vi "BIO_get_ssl.vi"(8 "error in (no error)":errorcluster, 11 "BIO in":refnum<class "BIO.lvclass">) -> (0 "error out":errorcluster, 2 "SSL out":refnum<class "SSL.lvclass">, 3 "BIO out":refnum<class "BIO.lvclass">)   [LabVIEW 2013, in "OpenSSL Socket.lvlib" / "BIO.lvclass"]
uses:
  BIO.lvclass
  SSL/SSL.lvclass
  SSL-Lib/SSL-Lib.lvclass/SSL-Lib.ctl
  BIO.lvclass/BIO.ctl
  SSL/SSL.lvclass/SSL.ctl
  SSL-Lib/Read Crypto Library Path.vi
  Read Handle.vi
  SSL/Write Handle.vi
  SSL-Lib/SSL-Lib.lvclass
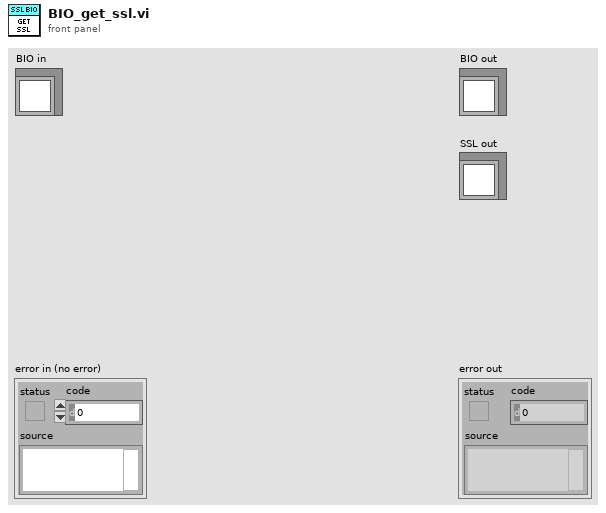
[diagram p1: front panel]
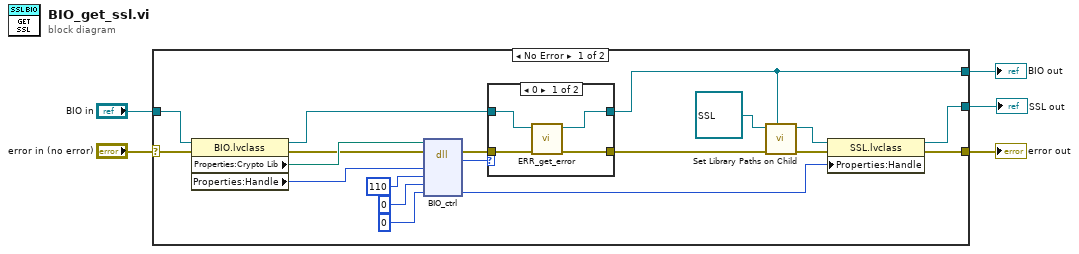
[diagram p0: block diagram]
diagram:
  n1 = case shown="No Error" "error in (no error)" {
    selector: "error in (no error)" -> [w20 w32]
    tunnel: [w7 w32] -> w4
    tunnel: [w10 w31] -> w2
    tunnel: "BIO in" -> [w21 w31]
    tunnel: [w6 _] -> w1
    frame No Error {
      n2 = property class="BIO.lvclass"(reference=w21, error in=w20) -> (reference out=w14:refnum<class "BIO.lvclass">, error out=w17:errorcluster, "Properties:Crypto Lib"=w19:path, "Properties:Handle"=w18:u64)
      n3 = dll-call lib="C:/Program Files (x86)/National Instruments/Shared/nissl/NIlibeay32.dll" fn="BIO_ctrl"(path in=w19, error in=w17, "BIO"=w18, "cmd"=110, "larg"=0, "parg"=u64 0 ("*SSL")) -> (error out=w15:errorcluster, "return type"=w16:i32, "parg"=w8:u64)  [unwired: 4 in, 1 out]
      n4 = case shown="0" w16 {
        tunnel: w15 -> [w28 w30]
        tunnel: [w25 w30] -> w13
        tunnel: w14 -> [w27 w29]
        tunnel: [w26 w29] -> w10
        frame 0 {
          n5 = call "ERR_get_error.vi"("error in (no error)"=w28, "SSL-Lib in"=w27) -> ("error out"=w25:errorcluster, "SSL-Lib out"=w26:refnum<class "BIO.lvclass">)  [unwired: 8 in]
        }
        frame Default {
        }
      }
      n6 = call-dynamic "Set Library Paths on Child.vi"(7:"SSL-Lib in"=w10, "error in (no error)"=w13, 11:"SSL-Lib in"=refnum<class "SSL.lvclass"> refnum ("SSL_Lib.lvlib:SSL.lvclass")) -> ("error out"=w12:errorcluster, "SSL-Lib out"=w9:refnum<class "SSL.lvclass">)  [unwired: 7 in]
      n7 = property class="SSL.lvclass"(reference=w9, error in=w12, "Properties:Handle"=w8) -> (reference out=w6:refnum<class "SSL.lvclass">, error out=w7:errorcluster)
    }
    frame Error {
    }
  }
  "error out" <- w4
  "BIO out" <- w2
  "SSL out" <- w1
